vi "PrepareHWI.vi"(8 "error in (no error)":errorcluster, 9 "Master Device in":refnum<class "Master Device.lvclass">, 10 "Current Variables":T1[](array[typedef]), 11 "Device in":refnum<class "Device.lvclass">) -> (0 "error out":errorcluster, 2 "Master Device out":refnum<class "Master Device.lvclass">, 3 "Device out":refnum<class "Device.lvclass">)   [LabVIEW 2013, in "Device.lvclass"]
doc: "Prepare HWI will parse string table values to generate a hardware image for each device. This is now accomplished with two subVIs which child classes must override: PasreSWI.vi and RequestTrig.vi. \nBoth variables and user functions can be pre-registered! This makes setting variables optional."
uses:
  Device.lvclass
  TypeDefs/Active procedure variables.ctl
  Master Device/Master Device.lvclass
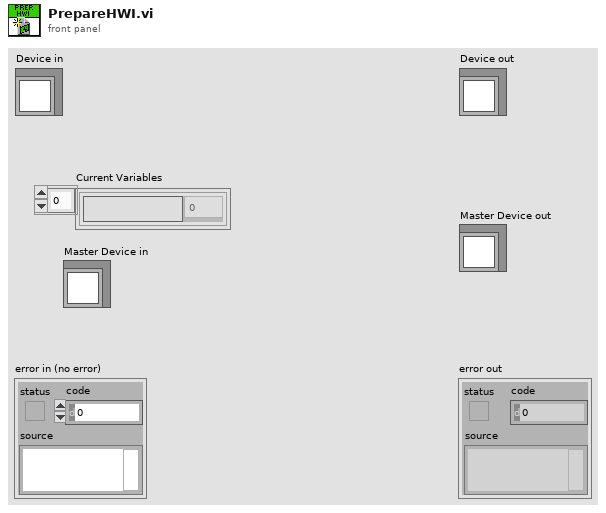
[diagram p1: front panel]
types:
  T1 = typedef "Active procedure variables.ctl" = cluster{"Procedure variable":string, "Value":dbl}
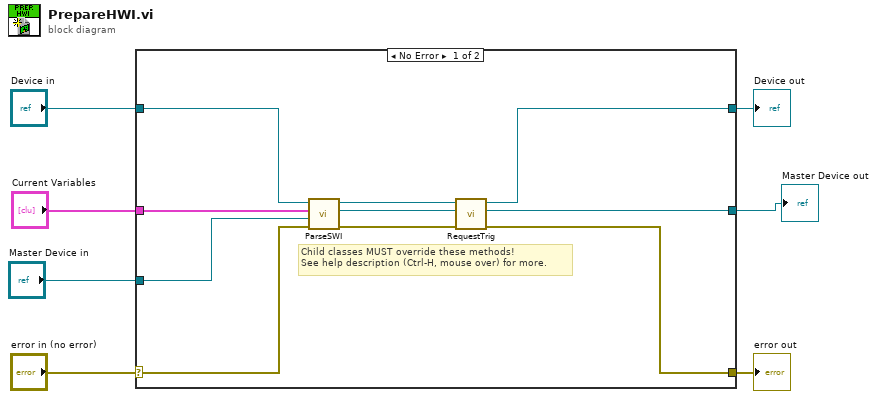
[diagram p0: block diagram]
diagram:
  n1 = case shown="No Error" "error in (no error)" {
    selector: "error in (no error)" -> [w14 w20]
    tunnel: [w13 w20] -> w6
    tunnel: [w8 w19] -> w4
    tunnel: "Device in" -> [w9 w19]
    tunnel: [w12 w18] -> w3
    tunnel: "Master Device in" -> [w11 w18]
    tunnel: "Current Variables" -> [w10 _]
    frame No Error {
      # "Child classes MUST override these methods!\nSee help description (Ctrl-H, mouse over) for more."
      n2 = call-dynamic "ParseSWI.vi"("error in (no error)"=w14, "Master Device in"=w11, "Current Variables"=w10, "Device in"=w9) -> ("error out"=w15:errorcluster, "Master Device out"=w16:refnum<class "Master Device.lvclass">, "Device out"=w17:refnum<class "Device.lvclass">)  [unwired: 5 in]
      n3 = call-dynamic "RequestTrig.vi"("error in (no error)"=w15, "Master Device in"=w16, "Device in"=w17) -> ("error out"=w13:errorcluster, "Master Device out"=w12:refnum<class "Master Device.lvclass">, "Device out"=w8:refnum<class "Device.lvclass">)  [unwired: 6 in]
    }
    frame Error {
      # "Wire the error cluster across even in the \"No Error\"\ncase so that warnings get propagated."
    }
  }
  "error out" <- w6
  "Device out" <- w4
  "Master Device out" <- w3
